vi "Debug.vi"() -> ()   [LabVIEW 2025]
panel:
  in  "System Definition File Path":path=path "C:/Users/Nick/Desktop/VCOM Config System Definition Utility/VeriStand Example Project/Example Project/Example Project.nivssdf"
  in  "Error in":errorcluster
  out "Signals Not Found in new VCOM Config":string[](array[string])
  out "error out":errorcluster
  in  "VCOM config file in":path=path "C:/Users/Public/Documents/National Instruments/NI-VCOM/configuration/Single_Point/CAN/VCOMConfig.xml"
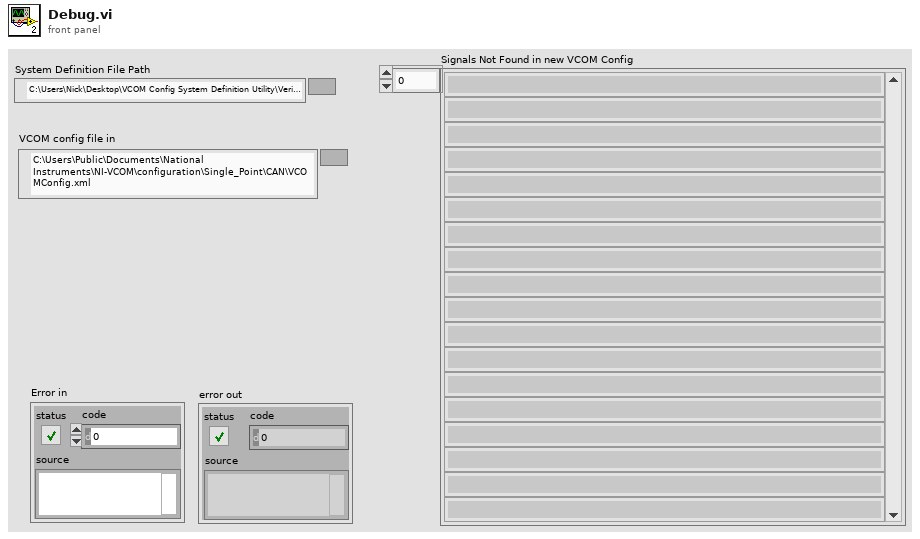
[diagram p1: front panel]
types:
  T1 = typedef "Vehicle Communication Toolkit.lvlib/RBS Signal.ctl" = cluster{"Name":string, "Description":string, "Unit":string, "Lower Limit":dbl, "Upper Limit":dbl, "Signal Type":enum32{"RE_BOOL", "RE_UINT8", "RE_INT8", "RE_UINT16", "RE_INT16", "RE_UINT32", "RE_INT32", "RE_UINT64", "RE_INT64", "RE_FLOAT32", "RE_FLOAT64", "RE_TEXT"}, "Text Table":cluster{"Text":string, "Min":dbl, "Max":dbl}[], "ReadOnly":bool, "Signal Dimensions":u32[], "Default Value":dbl, "Code Page":u32}
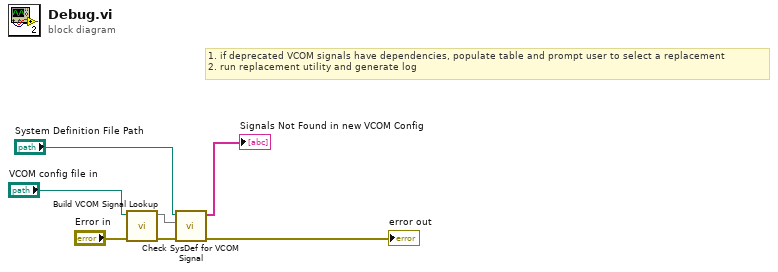
[diagram p0: block diagram]
diagram:
  # "1. if deprecated VCOM signals have dependencies, populate table and prompt user to select a replacement\n2. run replacement utility and generate log"
  n1 = call "Build VCOM Signal Lookup.vi"("Error in"="Error in", "VCOM config file in"="VCOM config file in") -> ("Error out"=w6:errorcluster, "VCOM Signal Map"=w7:map{string, T1})  [unwired: 7 in, 1 out]
  n2 = call "Check SysDef for VCOM Signal.vi"("error in (no error)"=w6, "VCOM Signal Map In"=w7, "System Definition File Path"="System Definition File Path") -> ("error out"=→"error out":errorcluster, "Signals Not Found in new VCOM Config"=→"Signals Not Found in new VCOM Config":string[])  [unwired: 6 in, 1 out]
